vi "Setup.vi"(8 "error in (no error)":errorcluster, 9 "Str Refnum":refnum<vi>, 10 "VI Reference":refnum<vi>, 11 "Msg_Error in":refnum<class "Msg_Error.lvclass">) -> (0 "error out":errorcluster, 2 "VI reference (dup)":refnum<vi>, 3 "Msg_Error out":refnum<class "Msg_Error.lvclass">)   [LabVIEW 2012, in "Msg_Error.lvlib" / "Msg_Error.lvclass"]
uses:
  Msg_Error.lvclass
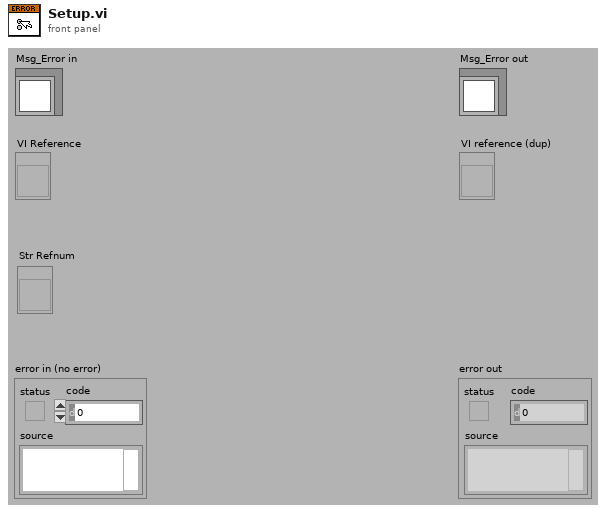
[diagram p1: front panel]
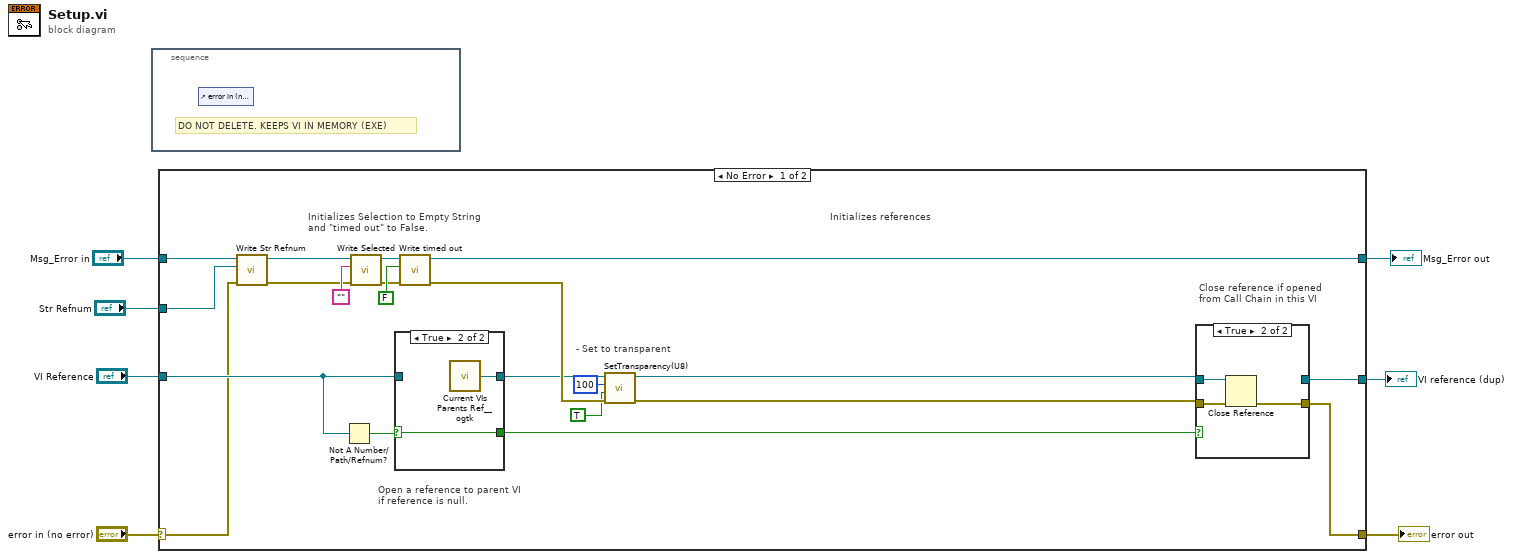
[diagram p0: block diagram]
diagram:
  n1 = stacked-sequence {
    frame #0 {
      # "DO NOT DELETE. KEEPS VI IN MEMORY (EXE)"
      n2 = control-ref of="error in (no error)"() -> ()  [unwired: 1 out]
    }
  }
  n3 = case shown="No Error" "error in (no error)" {
    selector: "error in (no error)" -> [w9 w40]
    tunnel: [w16 w40] -> w4
    tunnel: [w23 w39] -> w5
    tunnel: "Msg_Error in" -> [w11 w39]
    tunnel: "VI Reference" -> [w20 w38]
    tunnel: [w17 w38] -> w3
    tunnel: "Str Refnum" -> [w12 _]
    frame No Error {
      # "Open a reference to parent VI\nif reference is null."
      # "Close reference if opened\nfrom Call Chain in this VI"
      # "Initializes references"
      # "Initializes Selection to Empty String\nand \"timed out\" to False."
      # "- Set to transparent"
      n4 = call-dynamic "Write Str Refnum.vi"("error in (no error)"=w9, "Str Refnum"=w12, "Dialog.lvclass in"=w11) -> ("error out"=w8:errorcluster, "Dialog.lvclass out"=w10:refnum<class "Msg_Error.lvclass">)  [unwired: 7 out]
      n5 = Not A Number/Path/Refnum?(number/path/refnum=w20) -> (NaN/Path/Refnum?=w21:bool)
      n6 = call-dynamic "Write Selected.vi"("error in (no error)"=w8, "Selected"="", "Dialog.lvclass in"=w10) -> ("error out"=w24:errorcluster, "Dialog.lvclass out"=w26:refnum<class "Msg_Error.lvclass">)  [unwired: 7 out]
      n7 = case shown="True" w21 {
        selector: w21 -> [w34 w36]
        tunnel: w20 -> [w35 _]
        tunnel: [w35 w37] -> w19
        tunnel: [w34 w36] -> w18
        frame False {
        }
        frame True {
          n8 = call <userlib>:"Current VIs Parents Ref__ogtk.vi"() -> ("Calling VI's Reference"=w37:refnum<vi>)  [unwired: 2 out]
        }
      }
      n9 = call-dynamic "Write timed out.vi"("error in (no error)"=w24, "timed out?"=FALSE, "Dialog.lvclass in"=w26) -> ("error out"=w22:errorcluster, "Dialog.lvclass out"=w23:refnum<class "Msg_Error.lvclass">)  [unwired: 7 out]
      n10 = call "SetTransparency(U8).vi"("error in"=w22, "Run VI Transparently (T)"=TRUE, "Transparency (%)"=u8 100, "VI Reference (calling VI)"=w19) -> ("error out"=w13:errorcluster, "dup VI Reference"=w14:refnum<vi>)  [unwired: 6 out]
      n11 = case shown="True" w18 {
        tunnel: w14 -> [w30 w33]
        tunnel: [w30 _] -> w17
        tunnel: w13 -> [w29 w32]
        tunnel: [w29 w31] -> w16
        frame False {
        }
        frame True {
          n12 = Close Reference(reference=w33, error in (no error)=w32) -> (error out=w31:errorcluster)
        }
      }
    }
    frame Error {
    }
  }
  "error out" <- w4
  "Msg_Error out" <- w5
  "VI reference (dup)" <- w3
